vi "extract central core for intensity.vi"() -> ()   [LabVIEW 2020]
uses:
  <vilib>/Math Plots/3D Math Plots/3D Surface/3D Surface XCtrl/3D Surface.xctl
  <vilib>/Math Plots/3D Math Plots/3D Surface/3D Surface Datatype/Public/Plot Helper (Vector).vi
  <vilib>/Math Plots/3D Math Plots/3D Surface/3D Surface Datatype/3D Surface Datatype.lvclass
panel:
  out "Core Image":T1(plugin-control)
  in  "Boolean":bool
  out "3D Surface":refnum<class "3D Plot Datatype.lvclass">[](xcontrol)
  in  "Intensity Graph colour palette":cluster{dbl, "Color Box":u32}[](array[cluster])=[{1000.0, "Color Box"=16714752}, {750.0, "Color Box"=15859456}, {500.0, "Color Box"=65289}, {250.0, "Color Box"=983260}, {0.0, "Color Box"=14418124}]
  out "output array":i16[](array[numeric])
  out "Intensity Graph 3":i16[][](graph)
  out "dim2_length":i32
  out "dim2_start":i32
  out "dim1_length":i32
  out "dim1_start":i32
  in  "Core extraction size":i32
  out "output variable 6":dbl
  out "output variable 5":dbl
  out "output variable 4":dbl
  out "output variable 3":dbl
  out "output variable 2":i32
  out "output variable":i32
  out "size(s)":i32[](array[numeric])
  out "Intensity Graph 2":i16[][](graph)
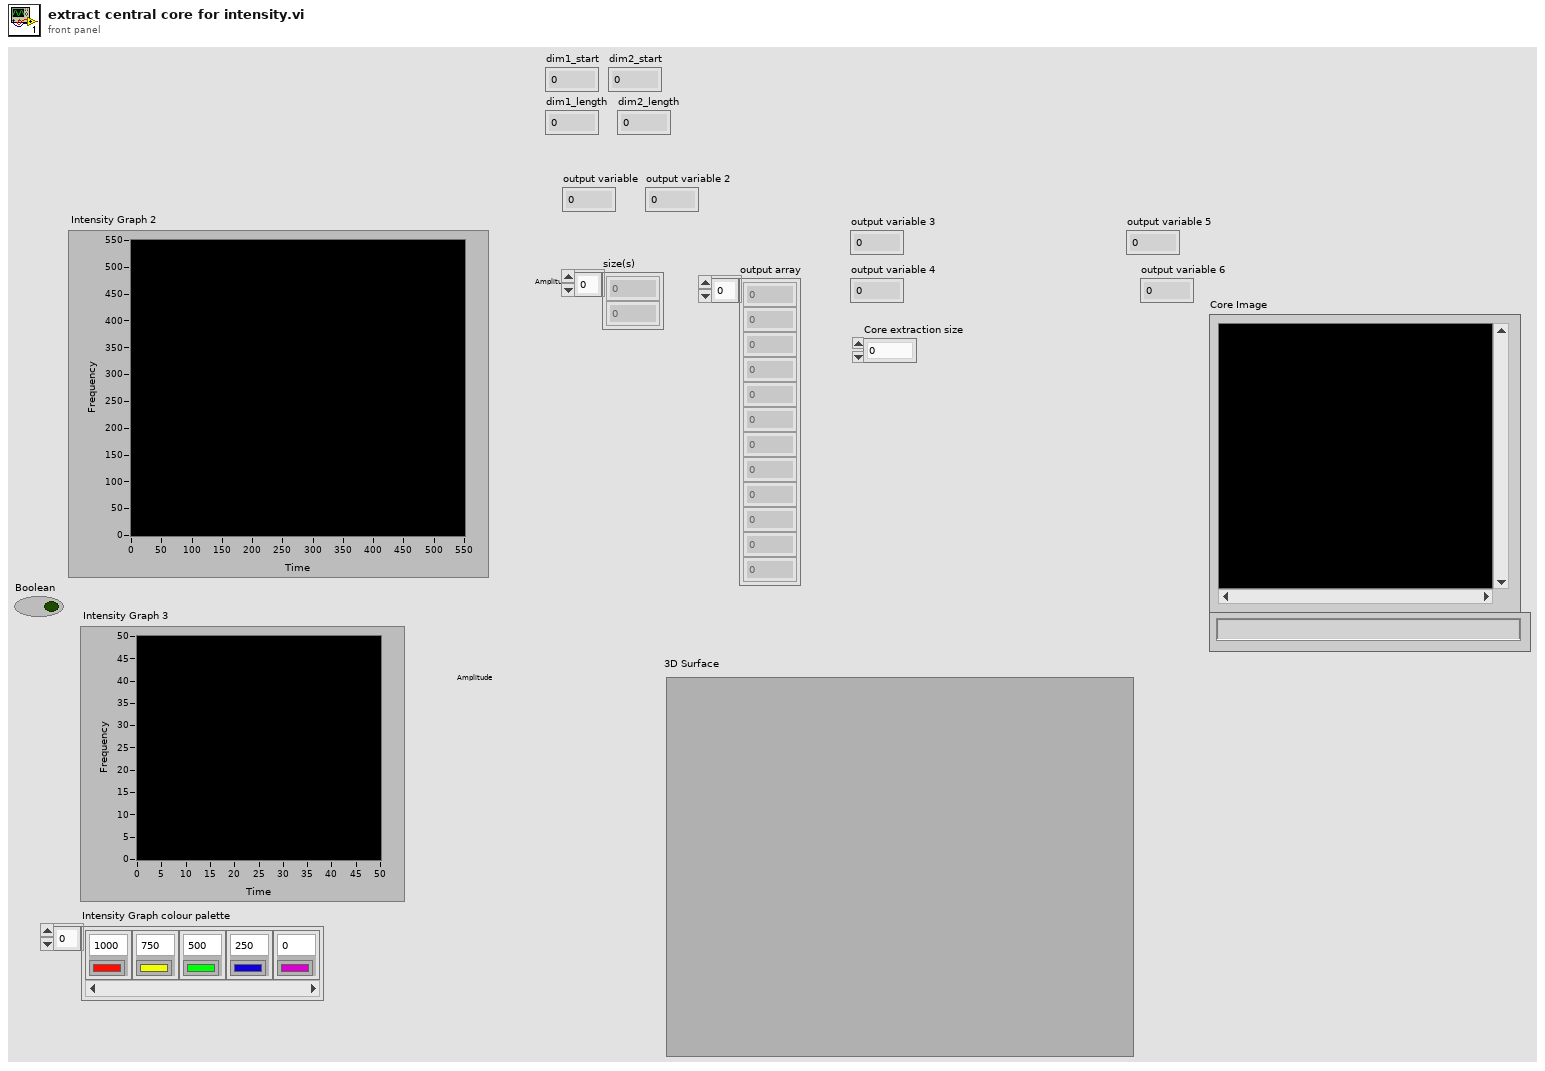
[diagram p1: front panel]
types:
  T1 = typedef "IMAQ Image.ctl" = refnum<image>
  T2 = typedef "Image Type" = u32
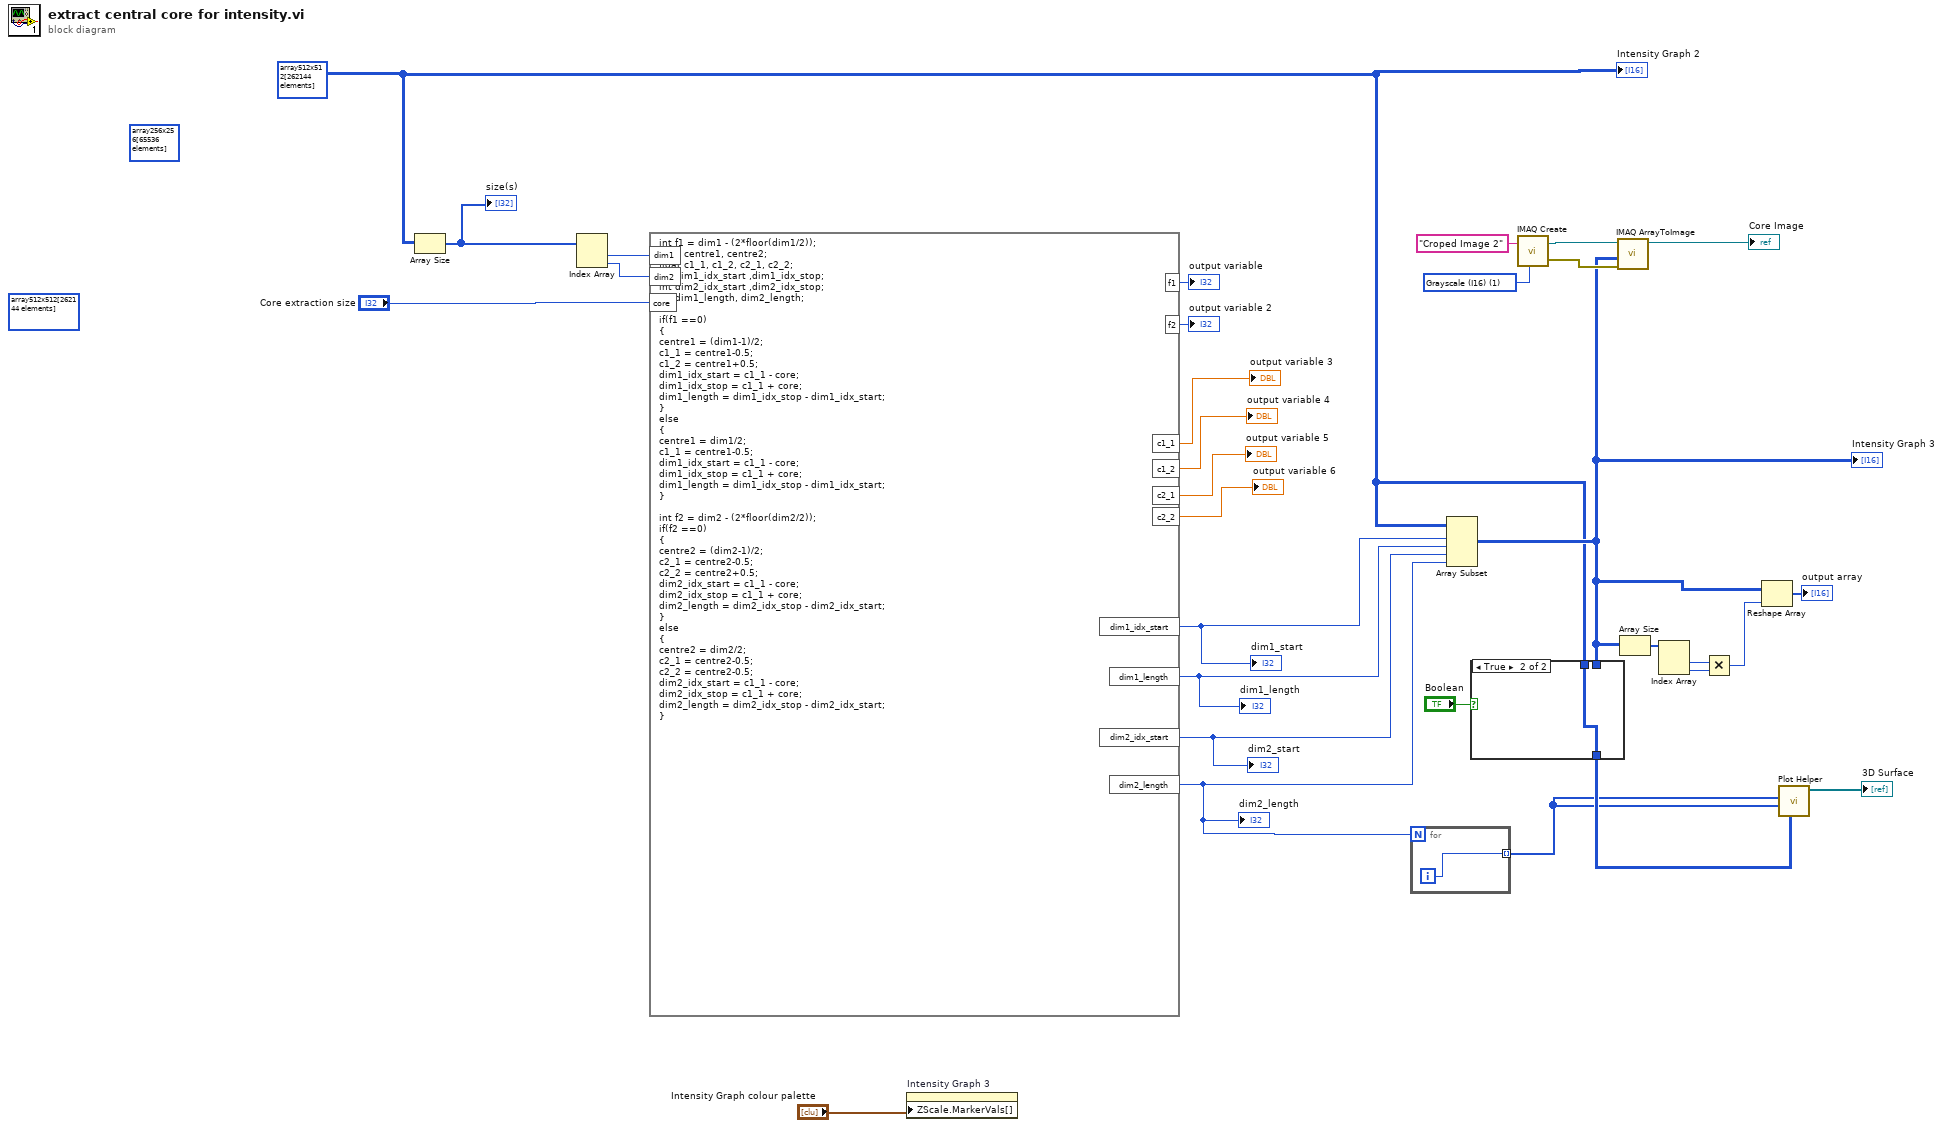
[diagram p0: block diagram]
diagram:
  w6 = T2 1 items=["Grayscale (U8)", "Grayscale (I16)", "Grayscale (SGL)", "Complex (CSG)", "RGB (U32)", "HSL (U32)", "RGB (U64)", "Grayscale (U16)"] ("Image Type")
  (unwired) i16[][] array256x256[65536 elements] ("Image Pixels (I16)")
  w1 = i16[][] array512x512[262144 elements] ("Image Pixels (I16)")
  (unwired) i16[][] array512x512[262144 elements] ("Intensity Graph 3")
  n1 = Array Size(array=w1) -> (size(s)=w31:i32[])
  "size(s)" <- w31
  n2 = Index Array(array=w31) -> (element #1=w30:i32, element #2=w29:i32)  [unwired: 2 in]
  n3 = formula code="int f1 = dim1 - (2*floor(dim1/2));\nfloat centre1, centre2;\nfloat c1_1, c1_2, c2_1, c2_2;\nint dim1_idx_start ,dim1_idx_stop;\nint dim2_idx_start ,dim2_idx_stop;\nint dim1_length, dim2_length;\n\nif(f1 ==0)\n{\ncentre1 = (dim1-1)/2;\nc1_1 = centre1-0.5;\nc1_2 = centre1+0.5;\ndim1_idx_start = c1_1 - core;\ndim1_idx_stop = c1_1 + core;\ndim1_length = dim1_idx_stop - dim1_idx_start;\n}\nelse\n{\ncentre1 = dim1/2;\nc1_1 = centre1-0.5;\ndim1_idx_start = c1_1 - core;\ndim1_idx_stop = c1_1 + core;\ndim1_length = dim1_idx_stop - dim1_idx_start;\n}\n\nint f2 = dim2 - (2*floor(dim2/2));\nif(f2 ==0)\n{\ncentre2 = (dim2-1)/2;\nc2_1 = centre2-0.5;\nc2_2 = centre2+0.5;\ndim2_idx_start = c1_1 - core;\ndim2_idx_stop = c1_1 + core;\ndim2_length = dim2_idx_stop - dim2_idx_start;\n}\nelse\n{\ncentre2 = dim2/2;\nc2_1 = centre2-0.5; \nc2_2 = centre2-0.5;\ndim2_idx_start = c1_1 - core;\ndim2_idx_stop = c1_1 + core;\ndim2_length = dim2_idx_stop - dim2_idx_start;\n}"("dim1"=w30, "dim2"=w29, "core"="Core extraction size") -> ("f1"=→"output variable":i32, "f2"=→"output variable 2":i32, "c1_1"=→"output variable 3":dbl, "c1_2"=→"output variable 4":dbl, "c2_1"=→"output variable 5":dbl, "c2_2"=→"output variable 6":dbl, "dim1_idx_start"=w21:i32, "dim1_length"=w20:i32, "dim2_idx_start"=w19:i32, "dim2_length"=w13:i32)
  "dim1_start" <- w21
  "dim1_length" <- w20
  "dim2_start" <- w19
  "dim2_length" <- w13
  n4 = property on="Intensity Graph 3" class="IntGraph (strict)"("ZScale.MarkerVals[]"="Intensity Graph colour palette") -> ()  [unwired: 2 in, 2 out]
  n5 = for {
    N: w13 -> [_]
    tunnel: [w32] -> w8 mode=indexing
    i -> [w32]
  }
  n6 = Array Subset(array=w1, index (row)=w21, length (row)=w20, index (col)=w19, length (col)=w13) -> (w2:i16[][])
  "Intensity Graph 3" <- w2
  n7 = case shown="True" "Boolean" {
    tunnel: w2 -> [w33 _]
    tunnel: [w33 w34] -> w10
    tunnel: w1 -> [_ w34]
    frame False {
    }
    frame True {
    }
  }
  n8 = call "IMAQ Create"("Image Name"="Croped Image 2", "Image Type"=w6) -> ("New Image"=w5:T1, "error out"=w4:errorcluster)  [unwired: 3 in]
  n9 = call "IMAQ ArrayToImage"("error in (no error)"=w4, "Image Pixels (I16)"=w2, "Image"=w5) -> ("Image Out"=→"Core Image":T1)  [unwired: 7 in, 1 out]
  n10 = Array Size(array=w2) -> (size(s)=w17:i32[])
  n11 = Index Array(array=w17) -> (element #1=w16:i32, element #2=w15:i32)  [unwired: 2 in]
  n12 = Multiply(x=w16, y=w15) -> (x*y=w14:i32)
  n13 = Reshape Array(w2, w14) -> (→"output array":i16[])
  n14 = call-poly <vilib>:"Plot Helper.vi"("z matrix"=w10, "y vector"=w8, "x vector"=w8) -> ("3D Plot lvclass Array out"=→"3D Surface":refnum<class "3D Plot Datatype.lvclass">[])  [unwired: 3 in, 5 out]
  "Intensity Graph 2" <- w1
